vi "get channels.vi"(11 "Scaling configuration in":refnum<class "Scaling configuration.lvclass">) -> (2 "channels":refnum<class "TBM channel.lvclass">[](array[class]), 3 "Scaling configuration out":refnum<class "Scaling configuration.lvclass">)   [LabVIEW 2013, in "Scaling configuration.lvclass"]
uses:
  Scaling configuration.lvclass
  <vilib>/NI/Tag Bus Module Framework/channel/TBM channel.lvclass
  Scaling configuration.lvclass/Scaling configuration.ctl
panel:
  out "size(s)":i32
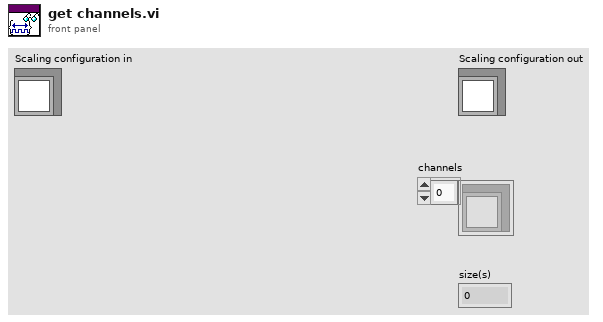
[diagram p1: front panel]
types:
  T1 = typedef "Scaling configuration.lvclass/scale data types.ctl" = enum16{"Double", "Single", "I64", "I32", "I16", "I8", "U64", "U32", "U16", "U8", "Boolean"}
  T2 = cluster{"mappings":cluster{"input channel":refnum<class "TBM channel.lvclass">, "output channel":refnum<class "TBM channel.lvclass">, "input data type":T1, "output data type":T1}[], "name":string}[]
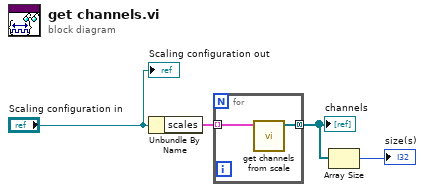
[diagram p0: block diagram]
diagram:
  n1 = Unbundle By Name("Scaling configuration in") -> ("scales"=w3:T2)
  n2 = for {
    tunnel: w3 -> [w6] mode=indexing
    tunnel: [w5] -> w2 mode=concatenating
    n3 = call "get channels from scale.vi"("Scale in"=w6) -> ("Channels"=w5:refnum<class "TBM channel.lvclass">[])  [unwired: 10 in]
  }
  "channels" <- w2
  n4 = Array Size(array=w2) -> (size(s)=→"size(s)":i32)
  "Scaling configuration out" <- "Scaling configuration in"
